vi "Async.Engine.Start.vi"(8 "error in (no error)":errorcluster, 11 "VS Inline Async API in":refnum<class "VS Inline Async API.lvclass">) -> (0 "error out":errorcluster, 3 "VS Inline Async API out":refnum<class "VS Inline Async API.lvclass">)   [LabVIEW 2027, in "VS Inline Async API.lvlib" / "VS Inline Async API.lvclass"]
uses:
  VS Inline Async API.lvclass
  VS Inline Async API.lvclass/VS Inline Async API.ctl
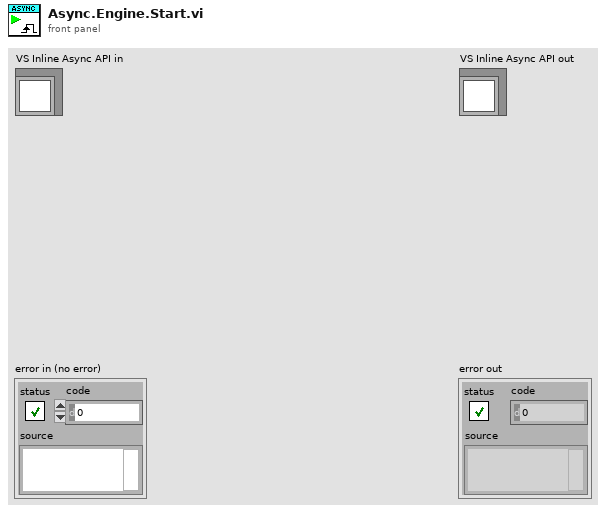
[diagram p1: front panel]
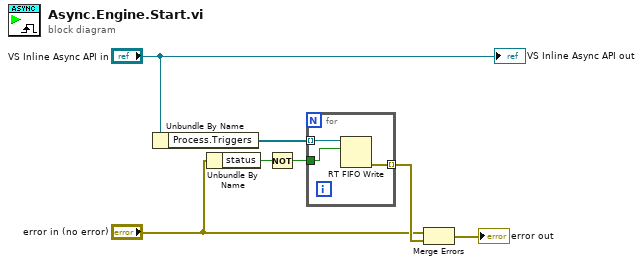
[diagram p0: block diagram]
diagram:
  n1 = Unbundle By Name("VS Inline Async API in") -> ("Process.Triggers"=w4:refnum<k33>[])
  n2 = Unbundle By Name("error in (no error)") -> ("status"=w2:bool)
  n3 = Not(x=w2) -> (.not. x?=w1:bool)
  n4 = for {
    tunnel: w4 -> [w10] mode=indexing
    tunnel: [w9] -> w6 mode=indexing
    tunnel: w1 -> [w8]
    n5 = RT FIFO Write(0:w10, 1:w8) -> (11:w9:errorcluster)  [unwired: 3 in, 3 out]
  }
  n6 = Merge Errors("error in (no error)", w6) -> (→"error out":errorcluster)
  "VS Inline Async API out" <- "VS Inline Async API in"
